vi "GetNumberOfSteps.vi"(9 "Step":dbl, 10 "Min":dbl, 11 "Max":dbl) -> (3 "unsigned 64bit integer":u64)   [LabVIEW 2021]
panel:
  out "Step (V) 2":dbl
  out "Min Voltage (V) 2":dbl
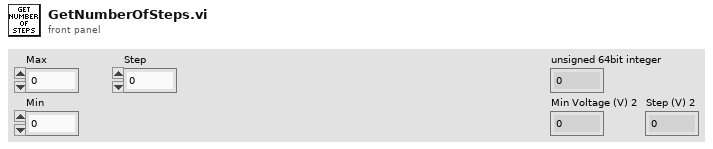
[diagram p1: front panel]
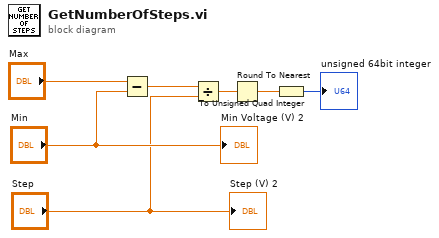
[diagram p0: block diagram]
diagram:
  n1 = Subtract(x="Max", y="Min") -> (x-y=w5:dbl)
  n2 = Divide(x=w5, y="Step") -> (x/y=w3:dbl)
  n3 = Round To Nearest(number=w3) -> (nearest integer value=w2:dbl)
  n4 = To Unsigned Quad Integer(1:w2) -> (0:→"unsigned 64bit integer":u64)
  "Min Voltage (V) 2" <- "Min"
  "Step (V) 2" <- "Step"
